vi "Write RewardAmount.vi"(8 "error in (no error)":errorcluster, 10 "RewardAmount":dbl, 11 "BehaviorClassification in":refnum<class "BehaviorClassification.lvclass">) -> (0 "error out":errorcluster, 3 "BehaviorClassification out":refnum<class "BehaviorClassification.lvclass">)   [LabVIEW 2010, in "BehaviorClassification.lvclass"]
uses:
  BehaviorClassification.lvclass
  BehaviorClassification.lvclass/BehaviorClassification.ctl
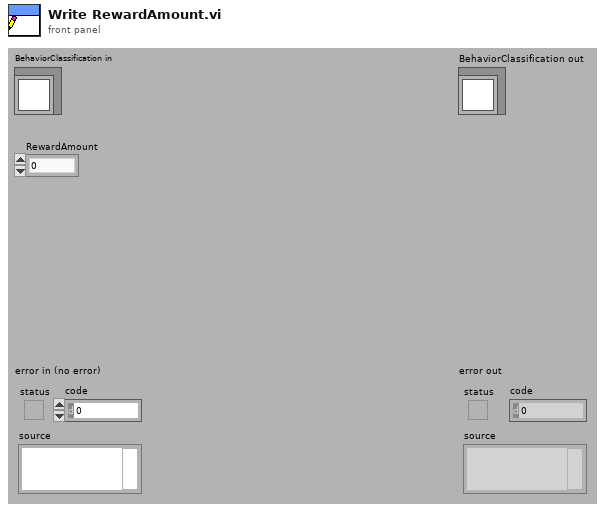
[diagram p1: front panel]
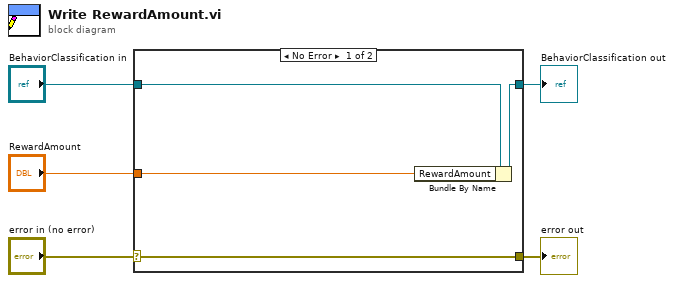
[diagram p0: block diagram]
diagram:
  n1 = case shown="No Error" "error in (no error)" {
    selector: "error in (no error)" -> [w9 w10]
    tunnel: [w9 w10] -> w4
    tunnel: [w7 w11] -> w2
    tunnel: "BehaviorClassification in" -> [w8 w11]
    tunnel: "RewardAmount" -> [w6 _]
    frame No Error {
      n2 = Bundle By Name(cluster=w8, "RewardAmount"=w6) -> (w7:refnum<class "BehaviorClassification.lvclass">)
    }
    frame Error {
    }
  }
  "error out" <- w4
  "BehaviorClassification out" <- w2
